vi "dlw_subPanel Worker.vi"(6 "Worker Alias":string="subPanel Worker", 7 "Caller in":refnum<class "Worker.lvclass">, 8 "error in":errorcluster, 10 "Initialization Data":T1, 11 "subPanel Worker in":refnum<class "subPanel Worker.lvclass">) -> (0 "error out":errorcluster, 3 "subPanel Worker out":refnum<class "subPanel Worker.lvclass">, 5 "dup Caller out":refnum<class "Worker.lvclass">)   [LabVIEW 2017, in "subPanel Worker.lvclass"]
doc: "This VI dynamically loads the Worker that owns this VI as a subWorker into <b>Caller</b>, and returns the Worker's object containing the Worker's Public Properties. Initialization data that is to be received by this Worker's <Initialize> MHL case can be wired to <b>Initialization Data</b>. The dynamically loaded Worker requires an alias ( <b>Worker Alias</b> ) which must be unique to the Worker it is called from. If a currently loaded subWorker exists with the same Alias, an error will be returned.\n\n<b>Note:</b> This VI can only be used from <b>within</b> a Worker's MHL. To load this Worker from an external LabVIEW application or from TestStand, please use an Asynchronous Launcher VI.\n---"
uses:
  subPanel Worker.lvclass
  C:/Program Files (x86)/National Instruments/LabVIEW 2017/vi.lib/addons/_Workers/Library/Classes/Worker/Worker.lvclass
  <vilib>/addons/_Workers/Library/Classes/Worker/Worker.lvclass
  Initialization Data.ctl
  Response Cases.ctl
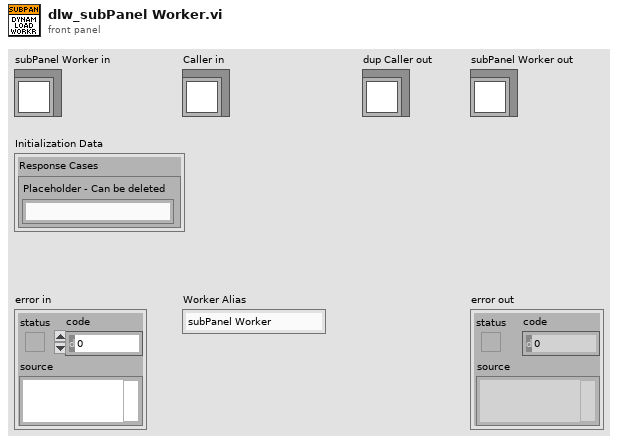
[diagram p1: front panel]
types:
  T1 = typedef "subPanel Worker.lvclass/Initialization Data.ctl" = cluster{"Response Cases":T2}
  T2 = typedef "subPanel Worker.lvclass/Response Cases.ctl" = cluster{"Placeholder - Can be deleted":string}
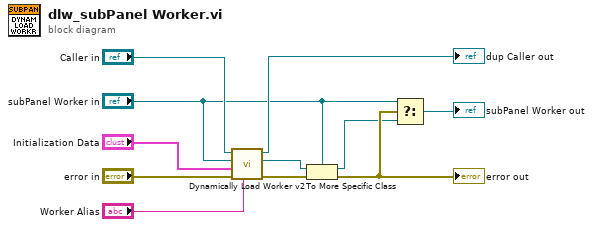
[diagram p0: block diagram]
diagram:
  n1 = call <vilib>:"Dynamically Load Worker v2.vi"("Worker Alias"="Worker Alias", "error in"="error in", "Initialization Data"="Initialization Data", "Worker to Dynamically Load"="subPanel Worker in", "Worker"="Caller in") -> ("error out"=w10:errorcluster, "Dynamically Loaded Worker out"=w5:refnum<class "Worker.lvclass">, "dup Worker out"=→"dup Caller out":refnum<class "Worker.lvclass">)  [unwired: 4 in]
  n2 = To More Specific Class(target class="subPanel Worker in", reference=w5, error in=w10) -> (specific class reference=w2:refnum<class "subPanel Worker.lvclass">, error out=w4:errorcluster)
  "error out" <- w4
  n3 = Select(t="subPanel Worker in", s=w4, f=w2) -> (s? t:f=→"subPanel Worker out":refnum<class "subPanel Worker.lvclass">)
